vi "EE_StopEmotivEpoc.vi"(8 "error in (no error)":errorcluster, 11 "EmotivEpocHeadsetControls in":refnum<class "EmotivEpocHeadsetControls.lvclass">) -> (0 "error out":errorcluster, 3 "EmotivEpocHeadsetControls out":refnum<class "EmotivEpocHeadsetControls.lvclass">)   [LabVIEW 2016, in "Emotiv Epoc.lvlib" / "EmotivEpocHeadsetControls.lvclass"]
uses:
  EmotivEpocHeadsetControls.lvclass
  <vilib>/Utility/error.llb/DialogType.ctl
  EmotivEpocHeadsetControls.lvclass/EmotivEpocHeadsetControls.ctl
panel:
  # "This VI is a part of BCI Design library, http://www.ru-bci.org \nCopyright © 2020, Sotnikov Peter, All rights reserved. License: GNU GPLv3"
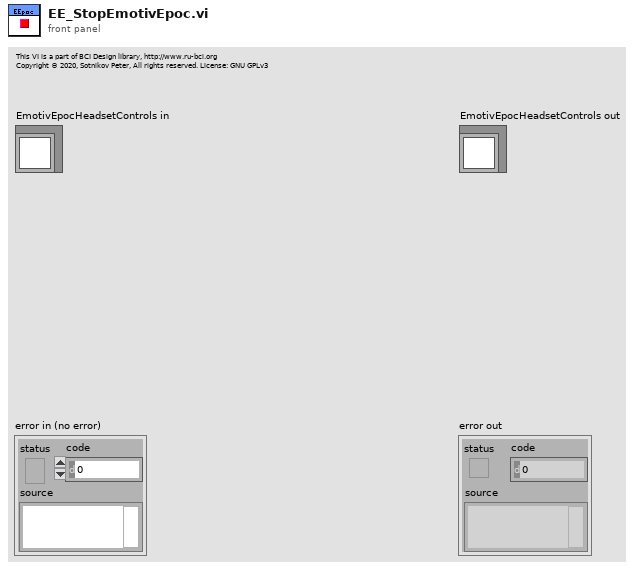
[diagram p1: front panel]
types:
  T1 = typedef "DialogType.ctl" = u16
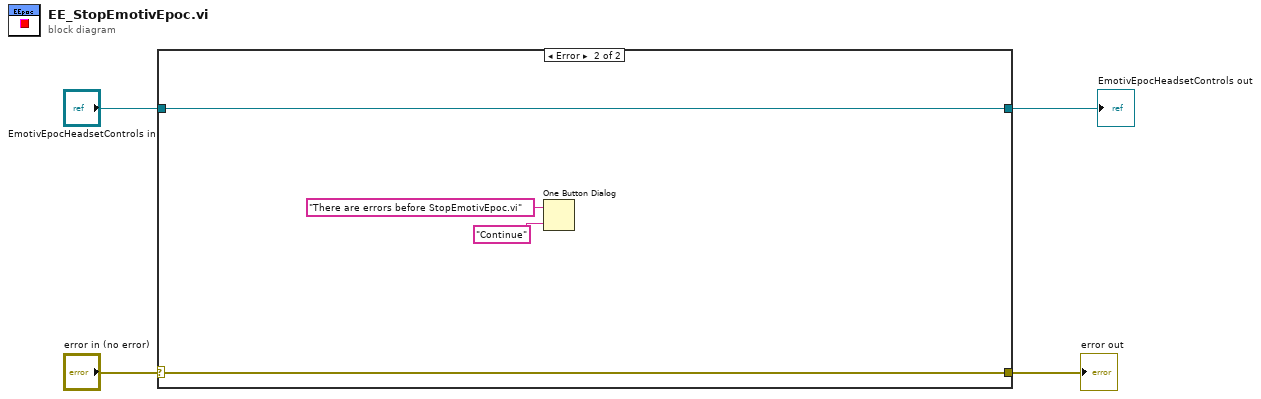
[diagram p0: block diagram]
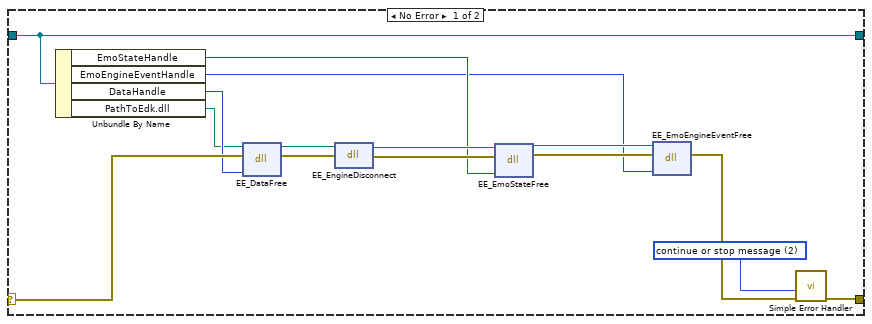
[diagram p2: hidden frame]
diagram:
  n1 = case shown="Error" "error in (no error)" {
    selector: "error in (no error)" -> [w12 w23]
    tunnel: [w7 w23] -> w3
    tunnel: [w13 w22] -> w1
    tunnel: "EmotivEpocHeadsetControls in" -> [w13 w22]
    frame No Error {
      w5 = T1 2 items=["no dialog", "OK message", "continue or stop message", "OK message + warnings", "continue/stop + warnings"] ("type of dialog (OK msg:1)")
      n2 = Unbundle By Name(w13) -> ("EmoStateHandle"=w9:i64, "EmoEngineEventHandle"=w8:i64, "DataHandle"=w11:i64, "PathToEdk.dll"=w10:path)
      n3 = dll-call lib="C:/Program Files/Emotiv Development Kit_v1.0.0.3-PREMIUM/edk.dll" fn="EE_DataFree"(path in=w10, error in=w12, "DataHandle"=w11) -> (path out=w18:path, error out=w19:errorcluster)  [unwired: 3 in]
      n4 = dll-call lib="C:/Program Files/Emotiv Development Kit_v1.0.0.3-PREMIUM/edk.dll" fn="EE_EngineDisconnect"(path in=w18, error in=w19) -> (path out=w16:path, error out=w17:errorcluster)  [unwired: 2 in]
      n5 = dll-call lib="C:/Program Files/Emotiv Development Kit_v1.0.0.3-PREMIUM/edk.dll" fn="EE_EmoStateFree"(path in=w16, error in=w17, "EmoStateHandle"=w9) -> (path out=w14:path, error out=w15:errorcluster)  [unwired: 3 in]
      n6 = dll-call lib="C:/Program Files/Emotiv Development Kit_v1.0.0.3-PREMIUM/edk.dll" fn="EE_EmoEngineEventFree"(path in=w14, error in=w15, "EmoEngineEventHandle"=w8) -> (error out=w6:errorcluster)  [unwired: 3 in, 1 out]
      n7 = call <vilib>:"Simple Error Handler.vi"("type of dialog (OK msg:1)"=w5, "error in (no error)"=w6) -> ("error out"=w7:errorcluster)  [unwired: 3 in, 4 out]
    }
    frame Error {
      n8 = One Button Dialog(message="There are errors before StopEmotivEpoc.vi", button name ("OK")="Continue") -> ()  [unwired: 1 out]
    }
  }
  "error out" <- w3
  "EmotivEpocHeadsetControls out" <- w1
